vi "TC560-Set Online.vi"(8 "error in":errorcluster, 10 "Online?":bool, 11 "VISA Resource Name In":refnum<visa-resource-name>) -> (0 "error out":errorcluster, 2 "Respond":string, 3 "VISA Resource Name Out":refnum<visa-resource-name>)   [LabVIEW 2018]
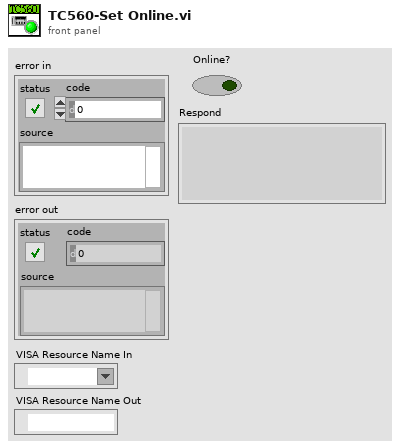
[diagram p1: front panel]
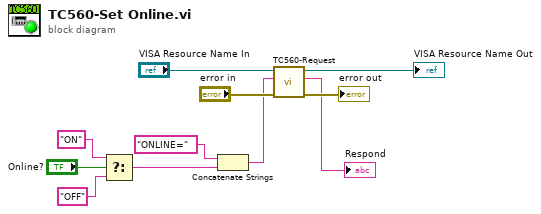
[diagram p0: block diagram]
diagram:
  n1 = Select(t="ON" ("write buffer"), s="Online?", f="OFF" ("write buffer")) -> (s? t:f=w7:string)
  n2 = Concatenate Strings("ONLINE=" ("write buffer"), w7) -> (w4:string)
  n3 = call "TC560-Request.vi"("error in"="error in", "Command"=w4, "VISA Resource Name In"="VISA Resource Name In") -> ("error out"=→"error out":errorcluster, "Respond"=→"Respond":string, "VISA Resource Name Out"=→"VISA Resource Name Out":refnum<visa-resource-name>)  [unwired: 6 in]
